vi "Split Factor Array.vi"(2 "Split character":string=":", 3 "STRING INPUT":string[](array[string])) -> (0 "FACTOR OUTPUT":sgl[](array[numeric]) format="%.7f", 1 "STRING OUTPUT":string[](array[string]))   [LabVIEW 2015]
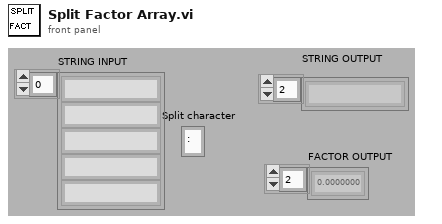
[diagram p1: front panel]
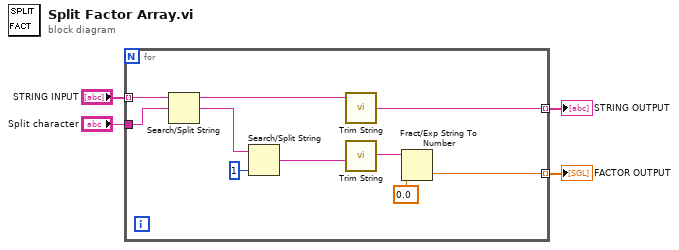
[diagram p0: block diagram]
diagram:
  n1 = for {
    tunnel: "STRING INPUT" -> [w14] mode=indexing
    tunnel: [w12] -> w4 mode=indexing
    tunnel: [w6] -> w2 mode=indexing
    tunnel: "Split character" -> [w5]
    n2 = Search/Split String(string=w14, search string/char (-)=w5) -> (substring before match=w13:string, match + rest of string=w11:string)  [unwired: 2 out]
    n3 = Search/Split String(string=w11, offset (0)=1) -> (match + rest of string=w9:string)  [unwired: 3 out]
    n4 = call "Trim String.vi"("inStr"=w13) -> ("outStr"=w12:string)
    n5 = call "Trim String.vi"("inStr"=w9) -> ("outStr"=w8:string)
    n6 = Fract/Exp String To Number(string=w8, default (0 dbl)=sgl 0.0) -> (number=w6:sgl)  [unwired: 3 out]
  }
  "STRING OUTPUT" <- w4
  "FACTOR OUTPUT" <- w2
